vi "sendMessage.vi"(8 "error in (no error)":errorcluster, 10 "message":string, 11 "MonoClientCommunicator in":refnum<class "MonoClientCommunicator.lvclass">) -> (0 "error out":errorcluster, 3 "MonoClientCommunicator out":refnum<class "MonoClientCommunicator.lvclass">)   [LabVIEW 2016, in "MonoClientCommunicator.lvclass"]
uses:
  MonoClientCommunicator.lvclass
  MonoClientCommunicator.lvclass/MonoClientCommunicator.ctl
  ts_labview_tcp/TCPClient/TCPClient.lvclass
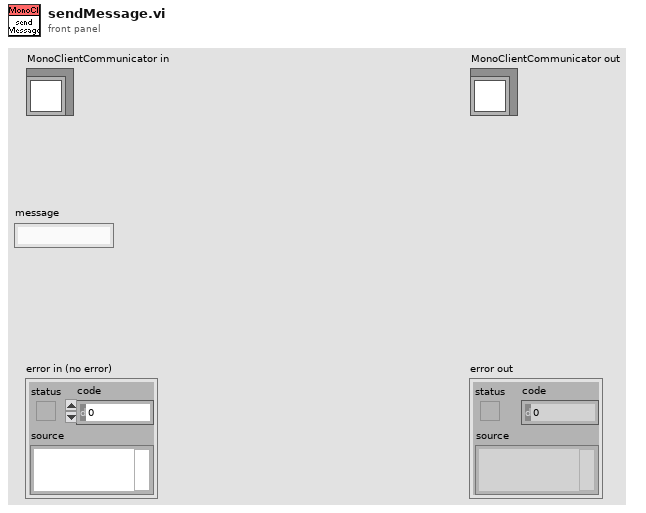
[diagram p1: front panel]
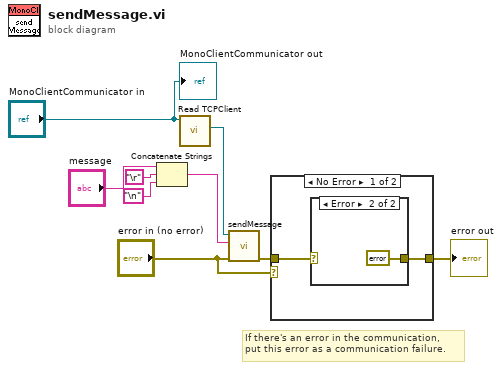
[diagram p0: block diagram]
diagram:
  # "If there's an error in the communication, \nput this error as a communication failure."
  n1 = Concatenate Strings("message", "\r", "\n") -> (w5:string)
  n2 = call "Read TCPClient.vi"("MonoClient in"="MonoClientCommunicator in") -> ("TCPClient.lvclass"=w4:refnum<class "TCPClient.lvclass">)  [unwired: 8 in, 2 out]
  n3 = call-dynamic "sendMessage.vi"("error in (no error)"="error in (no error)", "String"=w5, "TCPClient in"=w4) -> ("error out"=w3:errorcluster)  [unwired: 7 in, 1 out]
  n4 = case shown="No Error" "error in (no error)" {
    tunnel: w3 -> [w11 w14]
    tunnel: [w10 w14] -> w2
    frame No Error {
      n5 = case shown="Error" w11 {
        selector: w11 -> [w12 _]
        tunnel: [w12 errorcluster {"status"=TRUE, "code"=8204, "source"="Monochromator Controller not responding"} ("error IO")] -> w10
        frame No Error {
        }
        frame Error {
        }
      }
    }
    frame Error {
    }
  }
  "error out" <- w2
  "MonoClientCommunicator out" <- "MonoClientCommunicator in"
